vi "VI Server_Get Control Reference.vi"(7 "Label":string, 8 "error in":errorcluster, 9 "Single Instance (T)":bool=TRUE, 11 "VI Server Cluster":T1={"Labels"=["Label", "Size", "Font", "Heght", "Width", "Ledding Denominator", "Ledding Nominator", "Label Number", "Microstep Resolution", "X", "Y", "Z", "Italic?", "Underlined?"], "Refs"=[], "VI Ref"=refnum}) -> (0 "error out":errorcluster, 1 "Control Reference (Generic)":refnum<vi>, 2 "Found?":bool, 3 "VI Server Cluster.DUP":T1={"Labels"=["Label", "Size", "Font", "Heght", "Width", "Ledding Denominator", "Ledding Nominator", "Label Number", "Microstep Resolution", "X", "Y", "Z", "Italic?", "Underlined?"], "Refs"=[], "VI Ref"=refnum})   [LabVIEW 2020, in "VI Server Toolkit LV2013.lvlib"]
doc: "Returns \"generic\" (independent from the data type of the selected control) reference of the control, specified by label.\nUsed in cases when data type is too specific - graphs, clusters, enumerated, etc."
uses:
  VI Server Toolkit LV2013.lvlib
  VI Server_TypeDefs/VI Server_RefsCluster.ctl
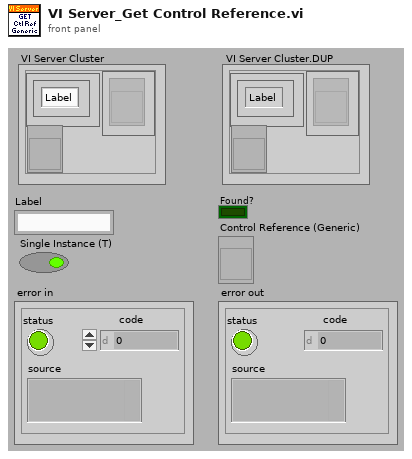
[diagram p1: front panel]
types:
  T1 = typedef "VI Server_RefsCluster.ctl" = cluster{"Labels":string[], "Refs":refnum<vi>[], "VI Ref":refnum<vi>}
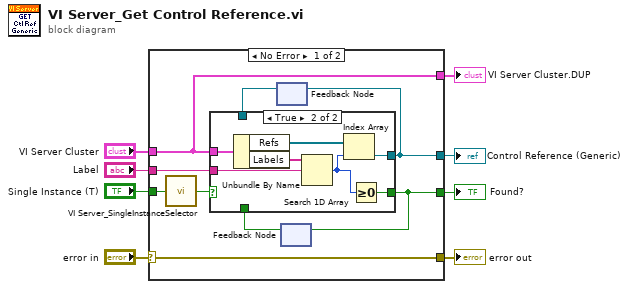
[diagram p0: block diagram]
diagram:
  n1 = case shown="No Error" "error in" {
    selector: "error in" -> [w16 w27]
    tunnel: "Label" -> [w17 _]
    tunnel: "VI Server Cluster" -> [w15 _]
    tunnel: [w16 w27] -> w8
    tunnel: [w12 _] -> w5
    tunnel: [w10 _] -> w3
    tunnel: [w15 _] -> w2
    tunnel: "Single Instance (T)" -> [w13 _]
    frame No Error {
      n2 = call "VI Server_SingleInstanceSelector.vi"("Single Instance (T)"=w13) -> ("Single Instance.OUT"=w14:bool)  [unwired: 6 in]
      n3 = feedback #1() -> (w11:refnum<vi>)  [unwired: 1 in]
      n4 = feedback #2() -> (w9:bool)  [unwired: 1 in]
      n5 = case shown="True" w14 {
        tunnel: w17 -> [_ w26]
        tunnel: [w18 w25] -> w10
        tunnel: w15 -> [_ w24]
        tunnel: [w19 w23] -> w12
        tunnel: w11 -> [w19 _]
        tunnel: w9 -> [w18 _]
        frame False {
        }
        frame True {
          n6 = Unbundle By Name(w24) -> ("Refs"=w21:refnum<vi>[], "Labels"=w22:string[])
          n7 = Search 1D Array(1D array=w22, element=w26) -> (index of element=w20:i32)  [unwired: 1 out]
          n8 = Index Array(array=w21, index=w20) -> (element=w23:refnum<vi>)
          n9 = Greater Or Equal To 0?(x=w20) -> (x >= 0?=w25:bool)
        }
      }
      n10 = feedback-in #1(w12) -> ()
      n11 = feedback-in #2(w10) -> ()
    }
    frame Error {
      n12 = call "VI Server_Empty VI Server Cluster.vi"() -> ()  [unwired: 7 in, 1 out]
    }
  }
  "error out" <- w8
  "Control Reference (Generic)" <- w5
  "VI Server Cluster.DUP" <- w2
  "Found?" <- w3
